vi "PressuresFP.vi"(10 "Array":waveform(dbl)[](array[waveform]), 11 "Pressures":dbl[](array[numeric])) -> ()   [LabVIEW 2023]
uses:
  <vilib>/Waveform/WDTOps.llb/WDT Number of Waveform Samples DBL.vi
panel:
  out "Waveform Graph":waveform(dbl)[](graph)
  out "Target PSI":dbl caption="PSI"
  out "PT 4":dbl caption="PSI"
  out "PT 3":dbl caption="PSI"
  out "PT 2":dbl caption="PSI"
  out "PT 1":dbl caption="PSI"
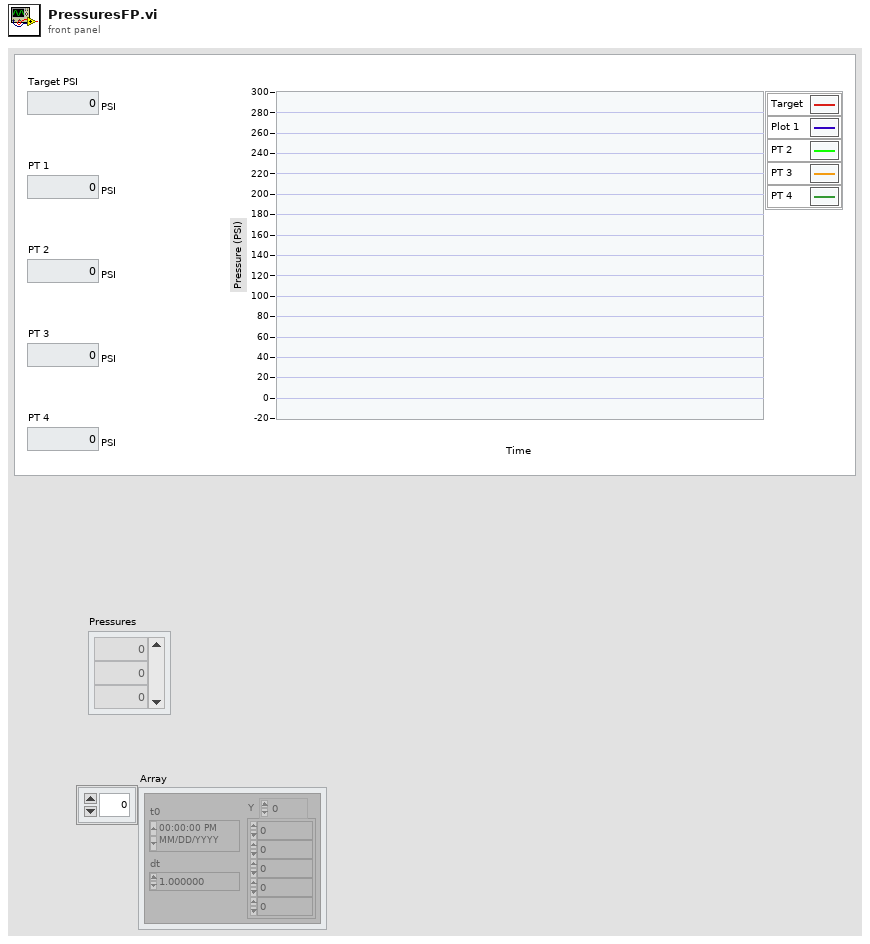
[diagram p1: front panel]
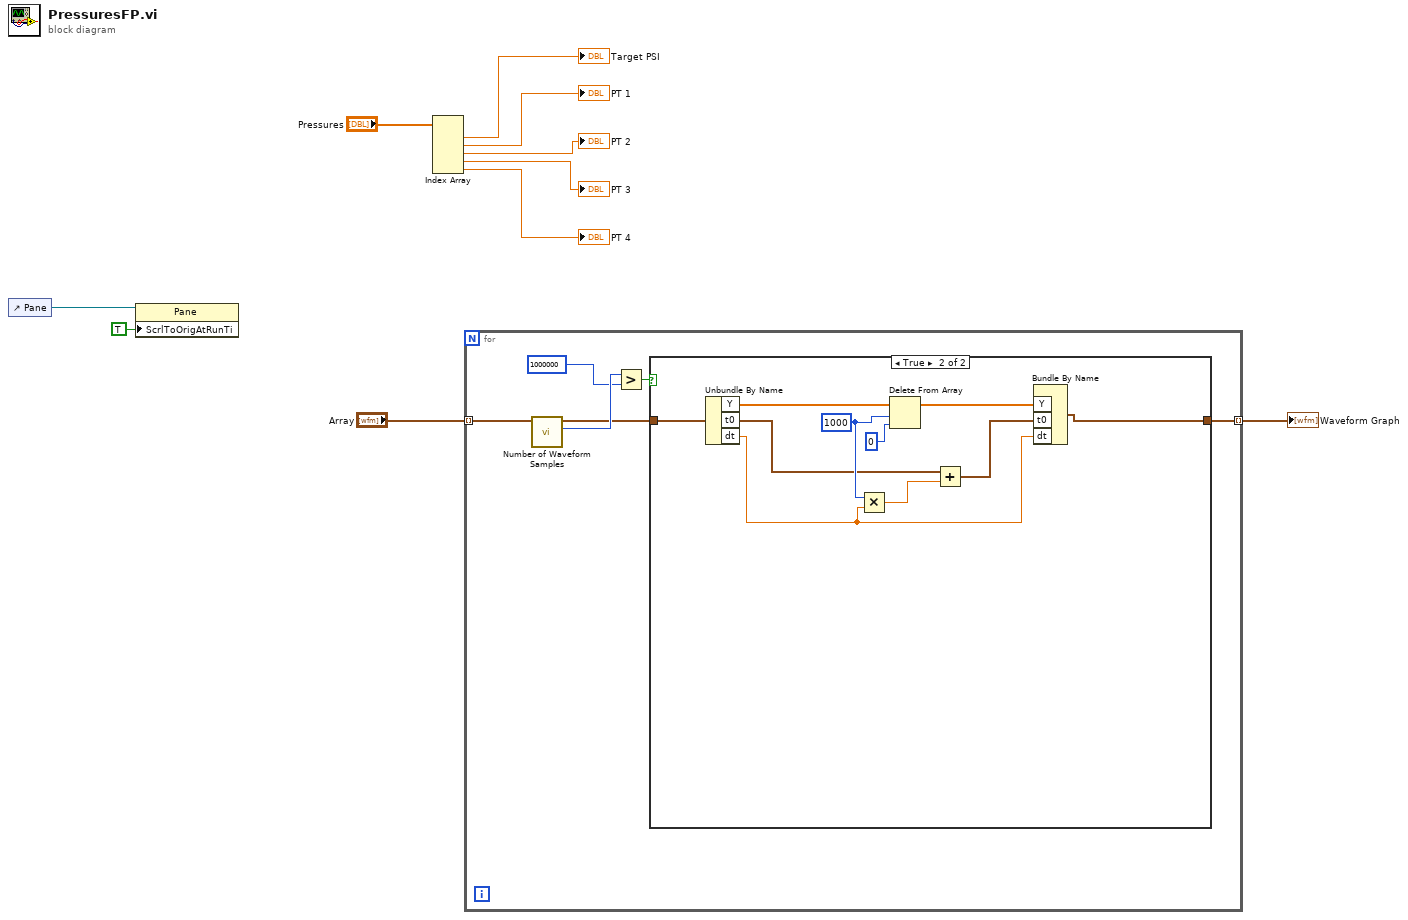
[diagram p0: block diagram]
diagram:
  n1 = control-ref of="Pane"() -> (w10:refnum<vi>)
  n2 = property class="Pane"(reference=w10, "ScrlToOrigAtRunTi"=TRUE ("Scroll To Origin At Run Time")) -> ()  [unwired: 1 in, 2 out]
  n3 = Index Array(array="Pressures") -> (element #1=→"Target PSI":dbl, element #2=→"PT 1":dbl, element #3=→"PT 2":dbl, element #4=→"PT 3":dbl, element #5=→"PT 4":dbl)  [unwired: 5 in]
  n4 = for {
    tunnel: "Array" -> [w13] mode=indexing
    tunnel: [w11] -> w1 mode=indexing
    n5 = call-poly <vilib>:"Number of Waveform Samples.vi"("waveform in"=w13) -> ("number of samples"=w15:i32, "waveform out"=w12:waveform(dbl))  [unwired: 8 in, 1 out]
    n6 = Greater?(x=w15, y=1000000) -> (0:w16:bool)
    n7 = case shown="True" w16 {
      tunnel: w12 -> [w17 w21]
      tunnel: [w17 w19] -> w11
      frame False {
      }
      frame True {
        w25 = 1000 ("length")
        n8 = Unbundle By Name(w21) -> ("Y"=w27:dbl[], "t0"=w24:timestamp, "dt"=w18:dbl)
        n9 = Multiply(x=w25, y=w18) -> (x*y=w23:dbl)
        n10 = Delete From Array(array=w27, length=w25, index=0) -> (array with subset deleted=w22:dbl[])  [unwired: 1 out]
        n11 = Add(x=w24, y=w23) -> (x+y=w20:timestamp)
        n12 = Bundle By Name("Y"=w22, "t0"=w20, "dt"=w18) -> (w19:waveform(dbl))  [unwired: 1 in]
      }
    }
  }
  "Waveform Graph" <- w1
